vi "add_TwistStamped_roslv.vi"(5 "Twist":T1, 6 "Stamp":cluster{"frame_id":string, "reset seq?":bool}, 7 "msg in":string) -> (3 "msg out":string)   [LabVIEW 2014]
doc: "Flattens a twist stamped into a message"
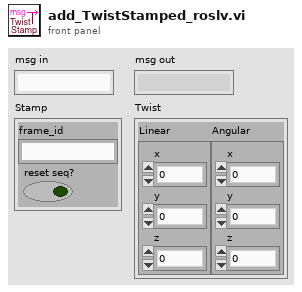
[diagram p1: front panel]
types:
  T1 = cluster{"Linear":cluster{"x":dbl, "y":dbl, "z":dbl}, "Angular":cluster{"x":dbl, "y":dbl, "z":dbl}}
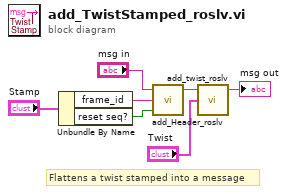
[diagram p0: block diagram]
diagram:
  # "Flattens a twist stamped into a message"
  n1 = Unbundle By Name("Stamp") -> ("frame_id"=w2:string, "reset seq?"=w1:bool)
  n2 = call "add_Header_roslv.vi"("reset seq?"=w1, "frame_id"=w2, "msg in"="msg in") -> ("msg out"=w6:string)  [unwired: 2 in]
  n3 = call "add_twist_roslv.vi"("Twist"="Twist", "msg in"=w6) -> ("msg out"=→"msg out":string)  [unwired: 3 in]
